vi "s-rflipflop.vi"(2 "Reset":bool, 3 "Set":bool) -> (0 "~Q":bool, 1 "Q":bool)   [LabVIEW 2014]
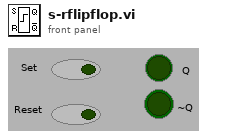
[diagram p1: front panel]
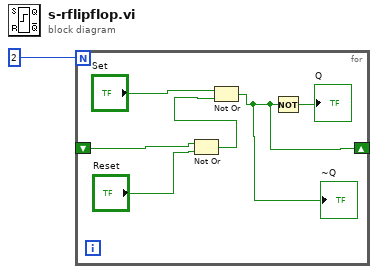
[diagram p0: block diagram]
diagram:
  n1 = for {
    N: 2 -> [_]
    shift-right: [w2] -> _
    shift-left: _ -> [w7]
    n2 = Not Or(1:"Reset", 2:w7) -> (0:w4:bool)
    n3 = Not Or(1:w4, 2:"Set") -> (0:w2:bool)
    "~Q" <- w2
    n4 = Not(x=w2) -> (.not. x?=→"Q":bool)
  }
